vi "DoE_Read_Standalone.vi"() -> (4 "all rows":dbl[][](array[numeric]) format="%0.3f", 8 "new file path (Not A Path if cancelled)":path)   [LabVIEW 2015]
uses:
  <vilib>/Utility/file.llb/Read From Spreadsheet File (DBL).vi
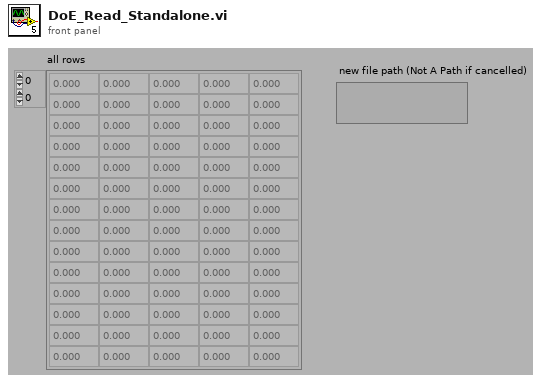
[diagram p1: front panel]
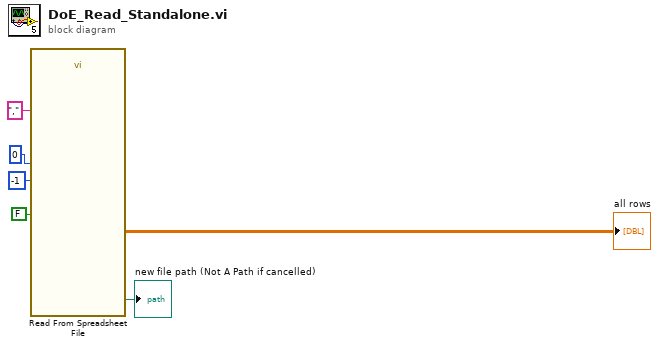
[diagram p0: block diagram]
diagram:
  n1 = call-poly <vilib>:"Read From Spreadsheet File.vi"("delimiter (\\t)"="," ("delimiter (\\t)"), "transpose (no:F)"=FALSE, "max characters/row  (no limit:0)"=0, "number of rows (all:-1)"=-1) -> ("all rows"=→"all rows":dbl[][], "new file path (Not A Path if cancelled)"=→"new file path (Not A Path if cancelled)":path)  [unwired: 3 in, 3 out]
